vi "CommonVIs_AttributeToDataType.vi"(1 "ClassInfo":T4[](array[typedef]), 2 "Array":string[](array[string])) -> (0 "Attributes":T1[](array[typedef]))   [LabVIEW 2020]
uses:
  CommonVIs_ClassNamePathType.ctl
  CommonVIs_AttributeType.ctl
  CommonVIs_AttributeDataType.ctl
  String/GDSString_AccessScopeModifierType.ctl
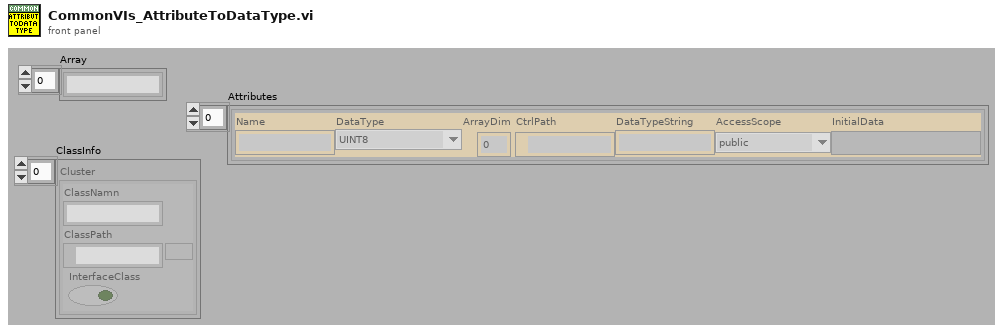
[diagram p1: front panel]
types:
  T1 = typedef "CommonVIs_AttributeType.ctl" = cluster{"Name":string, "DataType":T2, "ArrayDim":i32, "CtrlPath":path, "DataTypeString":string, "AccessScope":T3, "InitialData":variant}
  T2 = typedef "CommonVIs_AttributeDataType.ctl" = enum16{"UINT8", "INT8", "UINT16", "INT16", "UINT32", "INT32", "UINT64", "INT64", "SGL", "DBL", "EXT", "CSG", "CDB", "CXT", "TimeStamp", "STRING", "PATH", "BOOL", "ENUM", "RefNum", "VIRefNum", "LabVIEW Class", "Cluster", "Variant", "TypeDef", "Waveform", "LabVIEW Object", "Other", "void", "Set", "Map"}
  T3 = typedef "GDSString_AccessScopeModifierType.ctl" = enum16{"public", "private", "protected", "internal"}
  T4 = typedef "CommonVIs_ClassNamePathType.ctl" = cluster{"ClassNamn":string, "ClassPath":path, "InterfaceClass":bool}
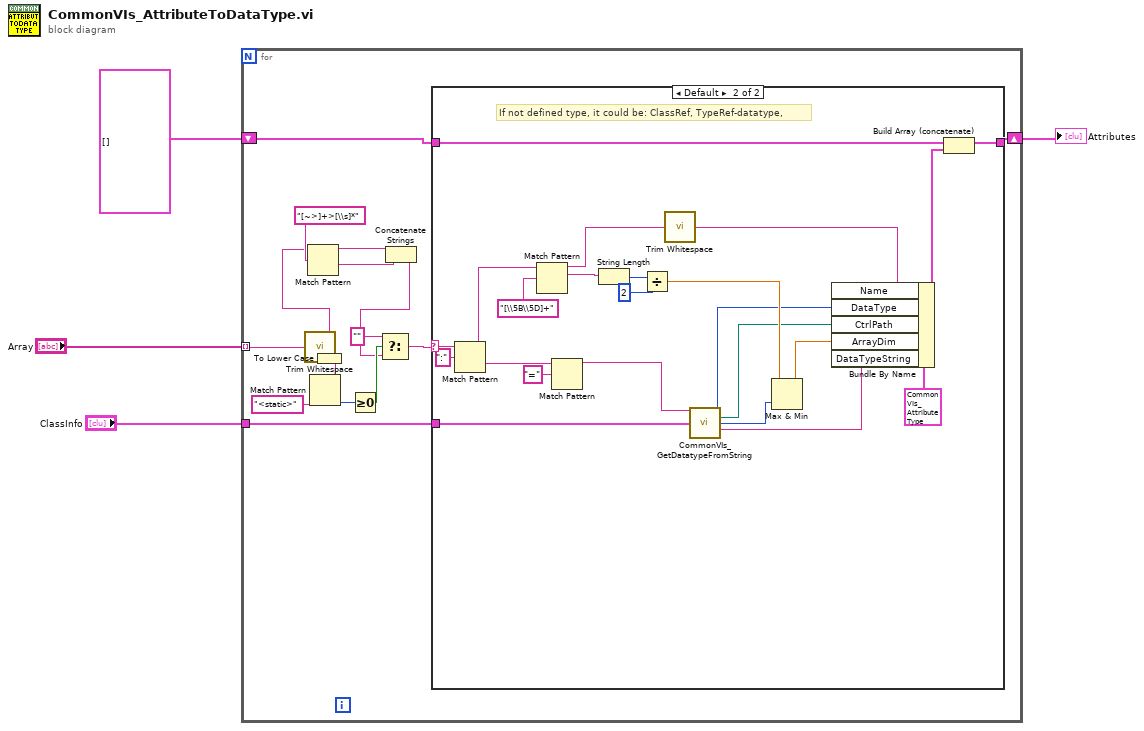
[diagram p0: block diagram]
diagram:
  n1 = for {
    tunnel: "Array" -> [w19] mode=indexing
    shift-right: [w17] -> w4
    shift-left: T1[] [] ("Attributes") -> [w18]
    tunnel: "ClassInfo" -> [w5]
    n2 = call <vilib>:"Trim Whitespace.vi"("string"=w19) -> ("trimmed string"=w13:string)  [unwired: 1 in]
    n3 = Match Pattern(string=w13, regular expression="[~>]+>[\\s]*") -> (before substring=w16:string, after substring=w15:string)  [unwired: 3 out]
    n4 = To Lower Case(string=w13) -> (all lower case string=w11:string)
    n5 = Match Pattern(string=w11, regular expression="<static>") -> (offset past match=w10:i32)  [unwired: 4 out]
    n6 = Greater Or Equal To 0?(x=w10) -> (x >= 0?=w9:bool)
    n7 = Concatenate Strings(w16, w15) -> (w8:string)
    n8 = Select(t="", s=w9, f=w8) -> (s? t:f=w6:string)
    n9 = case shown="Default" w6 {
      selector: w6 -> [_ w40]
      tunnel: w18 -> [w20 w43]
      tunnel: [w20 w42] -> w17
      tunnel: w5 -> [_ w21]
      frame "" {
      }
      frame Default {
        # "If not defined type, it could be: ClassRef, TypeRef-datatype,"
        n10 = Match Pattern(string=w40, regular expression=":") -> (before substring=w34:string, after substring=w36:string)  [unwired: 3 out]
        n11 = Match Pattern(string=w34, regular expression="[\\5B\\5D]+") -> (before substring=w33:string, match substring=w29:string)  [unwired: 3 out]
        n12 = Match Pattern(string=w36, regular expression="=") -> (before substring=w35:string)  [unwired: 4 out]
        n13 = String Length(string=w29) -> (length=w30:i32)
        n14 = Divide(x=w30, y=2) -> (x/y=w28:dbl)
        n15 = call <vilib>:"Trim Whitespace.vi"("string"=w33) -> ("trimmed string"=w38:string)  [unwired: 1 in]
        n16 = call "CommonVIs_GetDatatypeFromString.vi"("String"=w35, "Classes"=w21) -> ("AttributeDataType"=w24:T2, "ClassPath"=w23:path, "ArrayDimensions"=w27:i32, "DataTypeAsString(Array,default values removed)"=w25:string)  [unwired: 9 in, 1 out]
        n17 = Max & Min(x=w28, y=w27) -> (max(x,y)=w26:dbl)  [unwired: 1 out]
        n18 = Bundle By Name(cluster=T1 {"Name"="", "DataType"=enum."UINT8", "ArrayDim"=0, "CtrlPath"=path "", "DataTypeString"="", "AccessScope"=enum."public", "InitialData"=variant}, "Name"=w38, "DataType"=w24, "CtrlPath"=w23, "ArrayDim"=w26, "DataTypeString"=w25) -> (w22:T1)
        n19 = Build Array (concatenate)(w43, w22) -> (w42:T1[])
      }
    }
  }
  "Attributes" <- w4
